vi "选项启用写入.vi"(8 "error in (no error)":errorcluster caption="错误输入（无错误）", 10 "选项名称":cluster{"索引":i32, "enable":bool}, 11 "ScreenSwitching 输入":refnum<class "Screen Switching.lvclass">) -> (0 "error out":errorcluster caption="错误输出", 3 "ScreenSwitching 输出":refnum<class "Screen Switching.lvclass">)   [LabVIEW 2016, in "Screen Switching.lvlib" / "Screen Switching.lvclass"]
uses:
  Screen Switching.lvclass
  Screen Switching.lvclass/Screen Switching.ctl
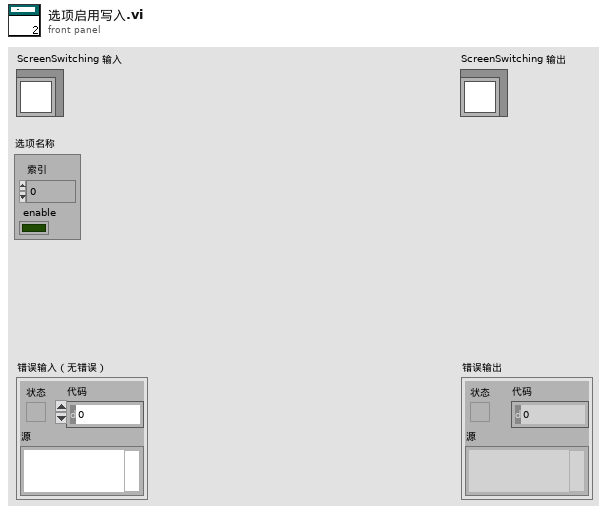
[diagram p1: front panel]
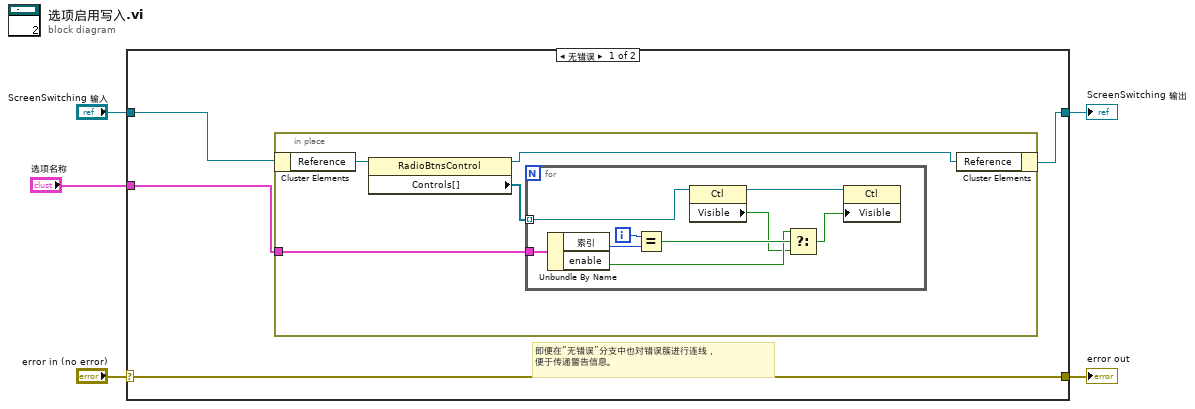
[diagram p0: block diagram]
diagram:
  n1 = case shown="无错误" "error in (no error)" {
    selector: "error in (no error)" -> [w9 w24]
    tunnel: [w9 w24] -> w4
    tunnel: [w6 w23] -> w2
    tunnel: "ScreenSwitching 输入" -> [w8 w23]
    tunnel: "选项名称" -> [w7 _]
    frame No Error {
      # "即便在“无错误”分支中也对错误簇进行连线，\n便于传递警告信息。"
      n2 = in-place {
        in-place-border: w7 -> [w11]
        n3 = in-place-cluster #1(w8) -> ("Reference"=w13:refnum<vi>)
        n4 = property class="RadioBtnsControl"(reference=w13) -> (reference out=w12:refnum<vi>, "Controls[]"=w10:refnum<vi>[])  [unwired: 1 in, 1 out]
        n5 = for {
          tunnel: w10 -> [w14] mode=indexing
          tunnel: w11 -> [w21]
          i -> [w20]
          n6 = Unbundle By Name(w21) -> ("索引"=w19:i32, "enable"=w17:bool)
          n7 = Equal?(x=w20, y=w19) -> (x = y?=w18:bool)
          n8 = property class="Ctl"(reference=w14) -> (reference out=w22:refnum<vi>, "Visible"=w16:bool)  [unwired: 1 in, 1 out]
          n9 = Select(t=w17, s=w18, f=w16) -> (s? t:f=w15:bool)
          n10 = property class="Ctl"(reference=w22, "Visible"=w15) -> ()  [unwired: 1 in, 2 out]
        }
        n11 = in-place-cluster #1("Reference"=w12) -> (w6:refnum<class "Screen Switching.lvclass">)
      }
    }
    frame Error {
    }
  }
  "error out" <- w4
  "ScreenSwitching 输出" <- w2
